vi "Draw Robot Trail.vi"(5 "Name":string) -> (1 "Scene:New Object":refnum<vi>)   [LabVIEW 2017]
uses:
  <vilib>/Utility/miscctls.llb/LV3DPointTypeDef.ctl
  <vilib>/picture/3D Picture Control/Object/Create Object (name).vi
  <vilib>/picture/3D Picture Control/NI_3D Picture Control.lvlib
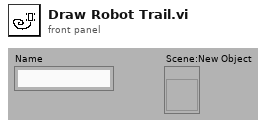
[diagram p1: front panel]
types:
  T1 = enum16{"Overall", "Per Primitive", "Per Vertex", "Binding Off"}
  T2 = typedef "LV3DPointTypeDef.ctl" = cluster{"X":sgl, "Y":sgl, "Z":sgl}
  T3 = enum16{"Points", "Lines", "Line Strip", "Line Loop", "Triangles", "Triangle Strip", "Triangle Fan", "Quads", "Quad Strip", "Polygon"}
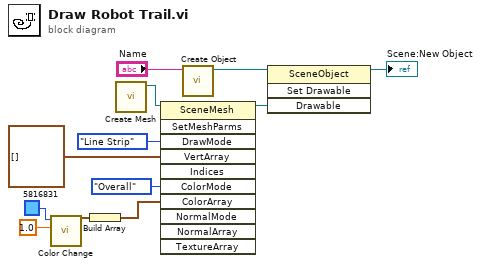
[diagram p0: block diagram]
diagram:
  n1 = call <vilib>:"Color Change.vi"("Alpha"=1.0, "Color"=u32 5816831) -> ("RGBA"=w3:cluster{"R":sgl, "G":sgl, "B":sgl, "A":sgl})  [unwired: 9 out]
  n2 = Build Array(w3) -> (w2:cluster{"R":sgl, "G":sgl, "B":sgl, "A":sgl}[])
  n3 = call <vilib>:"Create Mesh.vi"() -> ("New Mesh Refnum"=w8:refnum<vi>)  [unwired: 1 in, 10 out]
  n4 = invoke class="SceneMesh" method="SetMeshParms"(reference=w8, "DrawMode"=T3."Line Strip" ("Draw Mode"), "VertArray"=T2[] [] ("Vertex Array"), "ColorMode"=T1."Overall" ("Color Binding Mode"), "ColorArray"=w2) -> (reference out=w12:refnum<vi>)  [unwired: 6 in, 10 out]
  n5 = call-poly <vilib>:"Create Object.vi"("Name"="Name") -> ("Scene:New Object"=w11:refnum<vi>)  [unwired: 9 in, 1 out]
  n6 = invoke class="SceneObject" method="Set Drawable"(reference=w11, "Drawable"=w12) -> (reference out=→"Scene:New Object":refnum<vi>)  [unwired: 2 in, 3 out]
